vi "secParaChk.vi"(8 "error in":errorcluster, 9 "Row number":u32, 10 "Tbl Refnum in":refnum<vi>, 11 "Tree Refnum in":refnum<vi>) -> (0 "error out":errorcluster, 1 "Check result":string="√", 2 "Tbl Refnum out":refnum<vi>, 3 "Tree Refnum out":refnum<vi>)   [LabVIEW 2010]
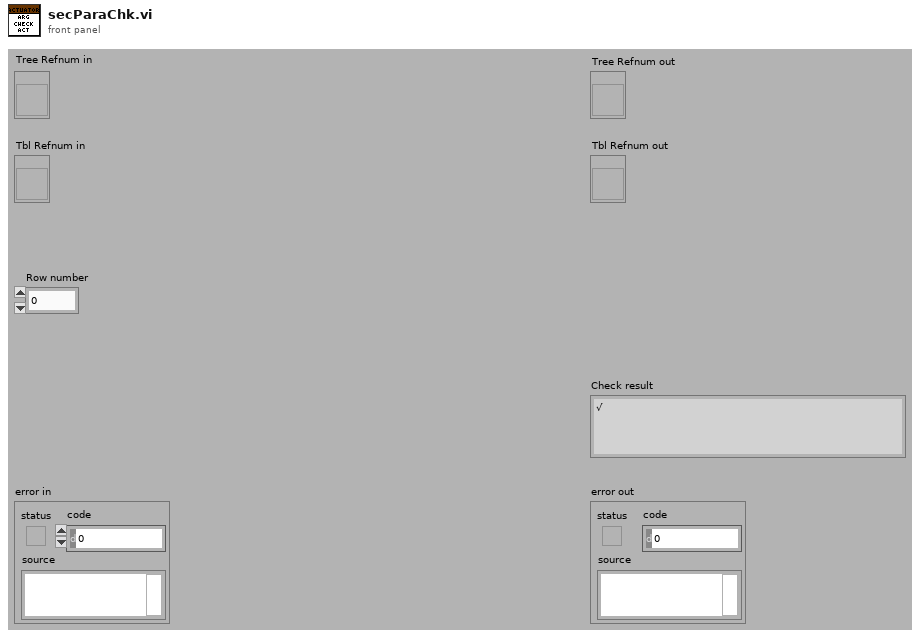
[diagram p1: front panel]
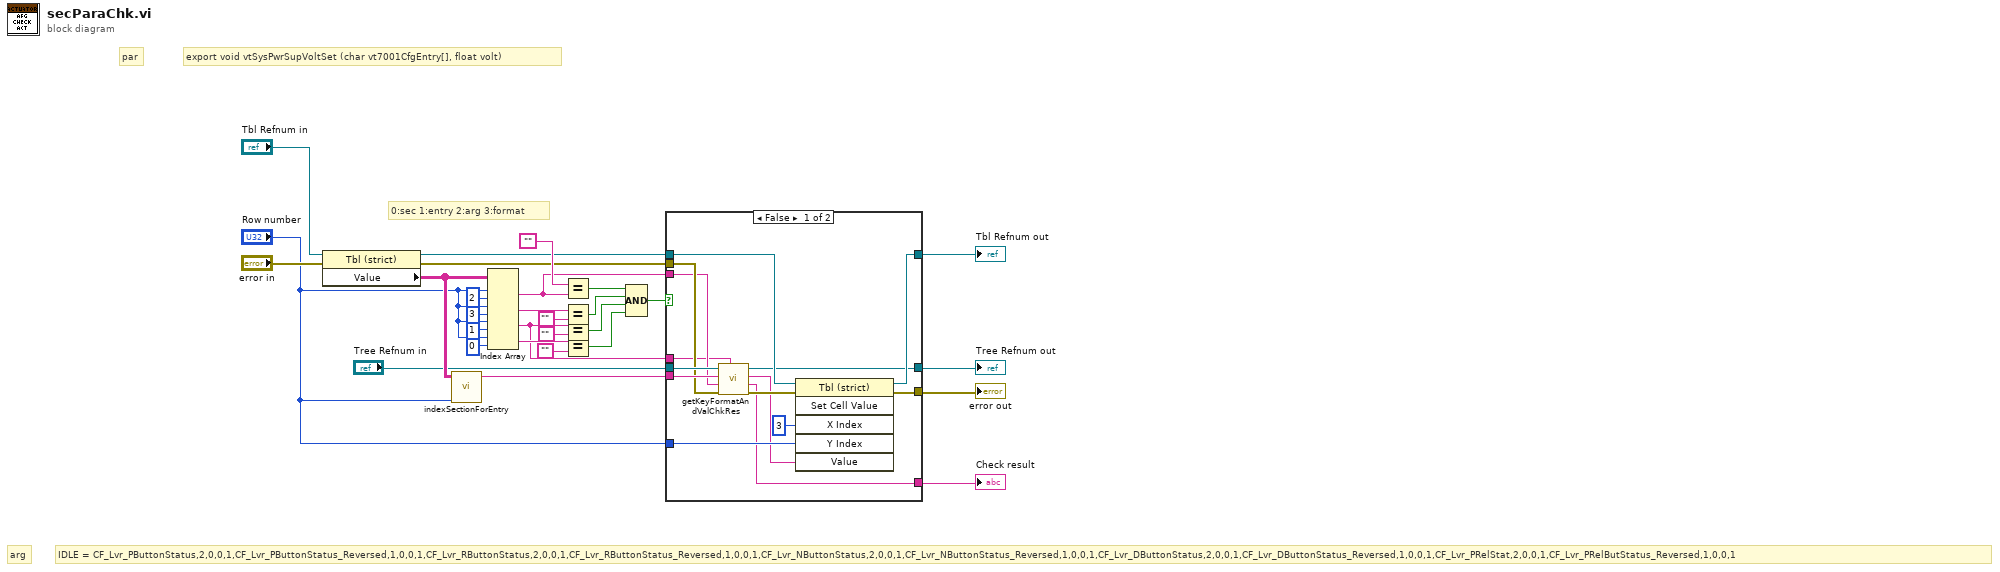
[diagram p0: block diagram]
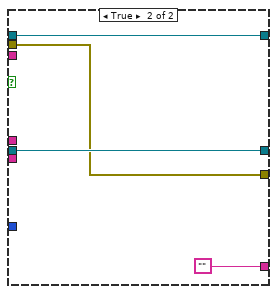
[diagram p2: hidden frame]
diagram:
  # "arg"
  # "par"
  # "0:sec 1:entry 2:arg 3:format"
  # "IDLE = CF_Lvr_PButtonStatus,2,0,0,1,CF_Lvr_PButtonStatus_Reversed,1,0,0,1,CF_Lvr_RButtonStatus,2,0,0,1,CF_Lvr_RButtonStatus_Reversed,1,0,0,1,CF_Lvr_NButtonStatus,2,0,0,1,CF_Lvr_NButtonStatus_Reversed,1,0,0,1,CF_Lvr_DButtonStatus,2,0,0,1,CF_Lvr_DButtonStatus_Reversed,1,0,0,1,CF_Lvr_PRelStat,2,0,0,1,CF_Lvr_PRelButStatus_Reversed,1,0,0,1"
  # "export void vtSysPwrSupVoltSet (char vt7001CfgEntry[], float volt)"
  n1 = property class="Tbl (strict)"(reference="Tbl Refnum in", error in="error in") -> (reference out=w15:refnum<vi>, error out=w16:errorcluster, "Value"=w26:string[][])
  n2 = call "indexSectionForEntry.vi"("rowNum"="Row number", "tbl"=w26) -> ("indexSection"=w18:string)  [unwired: 9 in]
  n3 = Index Array(array=w26, index (row) #1="Row number", index (col) #1=2 ("index (col)"), index (row) #2="Row number", index (col) #2=3 ("index (col)"), index (row) #3="Row number", index (col) #3=1 ("disabled index (col)"), index (row) #4="Row number", index (col) #4=0 ("disabled index (col)")) -> (element #1=w17:string, element #2=w24:string, element #3=w1:string, element #4=w4:string)
  n4 = Equal?(x="", y=w17) -> (x = y?=w22:bool)
  n5 = Equal?(x=w24, y="") -> (x = y?=w21:bool)
  n6 = Equal?(x=w1, y="") -> (x = y?=w8:bool)
  n7 = Equal?(x=w4, y="") -> (x = y?=w2:bool)
  n8 = Compound Arithmetic op=AND(w22, w21, w8, w2) -> (w20:bool)
  n9 = case shown="False" w20 {
    tunnel: "Tree Refnum in" -> [w43 w46]
    tunnel: w18 -> [w42 _]
    tunnel: w17 -> [w36 _]
    tunnel: w16 -> [w41 w45]
    tunnel: w15 -> [w40 w47]
    tunnel: "Row number" -> [w38 _]
    tunnel: [w34 w45] -> w14
    tunnel: [w33 w47] -> w13
    tunnel: [w32 w46] -> w12
    tunnel: [w31 ""] -> w11
    tunnel: w1 -> [w30 _]
    frame False {
      n10 = call "getKeyFormatAndValChkRes.vi"("entryName"=w30, "error in"=w41, "arg"=w36, "sec"=w42, "Tree Refnum in"=w43) -> ("error out"=w39:errorcluster, "Check result"=w31:string, "entryFormat"=w35:string, "Tree Refnum out"=w32:refnum<vi>)  [unwired: 3 in]
      n11 = invoke class="Tbl (strict)" method="Set Cell Value"(reference=w40, error in=w39, "X Index"=u32 3, "Y Index"=w38, "Value"=w35) -> (reference out=w33:refnum<vi>, error out=w34:errorcluster)  [unwired: 1 in, 4 out]
    }
    frame True {
    }
  }
  "Check result" <- w11
  "error out" <- w14
  "Tbl Refnum out" <- w13
  "Tree Refnum out" <- w12
